vi "Set Exclusions By Path.vi"(8 "error in (no error)":errorcluster, 10 "Path exclusions":T1={"Exclude files from vi.lib"=TRUE, "Exclude files from instr.lib"=TRUE, "Exclude files from user.lib"=TRUE}, 11 "NI_AB_API_Build in":refnum<class "NI_AB_API_Build.lvclass">) -> (0 "error out":errorcluster, 3 "NI_AB_API_Build out":refnum<class "NI_AB_API_Build.lvclass">)   [LabVIEW 2020, in "NI_AB_API_Build.lvclass"]
uses:
  <vilib>/AppBuilder/AB_API/Build/NI_AB_API_Build.lvclass
  <vilib>/AppBuilder/AB_API/common/AB_API Path Exclusions.ctl
  <vilib>/AppBuilder/AB_API/Build/NI_AB_API_Build.lvclass/NI_AB_API_Build.ctl
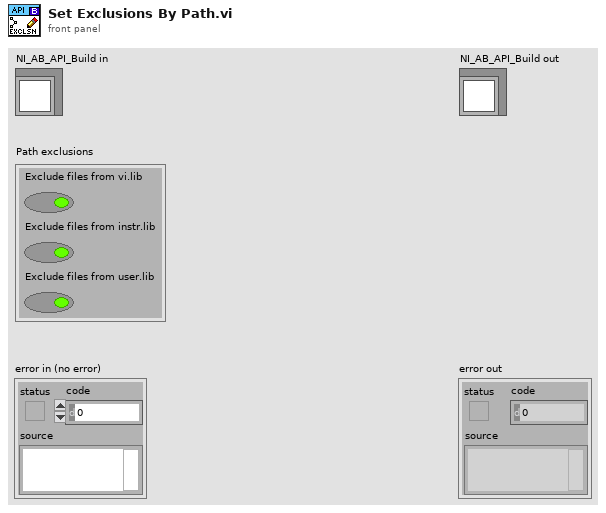
[diagram p1: front panel]
types:
  T1 = typedef "AB_API Path Exclusions.ctl" = cluster{"Exclude files from vi.lib":bool, "Exclude files from instr.lib":bool, "Exclude files from user.lib":bool}
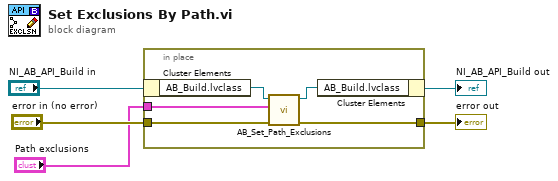
[diagram p0: block diagram]
diagram:
  n1 = in-place {
    in-place-border: "Path exclusions" -> [w10]
    in-place-border: "error in (no error)" -> [w9]
    in-place-border: [w8] -> w4
    n2 = in-place-cluster #1("NI_AB_API_Build in") -> ("AB_Build.lvclass"=w7:refnum<class "AB_Build.lvclass">)
    n3 = call <vilib>:"AB_Set_Path_Exclusions.vi"("error in (no error)"=w9, "Path exclusions"=w10, "Build in"=w7) -> ("error out"=w8:errorcluster, "Build out"=w6:refnum<class "AB_Build.lvclass">)  [unwired: 7 in]
    n4 = in-place-cluster #1("AB_Build.lvclass"=w6) -> (→"NI_AB_API_Build out":refnum<class "NI_AB_API_Build.lvclass">)
  }
  "error out" <- w4
